vi "Request Data.vi"(6 "Qualifier":string, 8 "error in":errorcluster, 9 "notifier":refnum<notifier>, 10 "Data to Send":string, 11 "Analog-Output in":refnum<class "Analog-Output.lvclass">) -> (0 "error out":errorcluster, 3 "Analog-Output out":refnum<class "Analog-Output.lvclass">)   [LabVIEW 2019, in "Analog-Output.lvlib" / "Analog-Output.lvclass"]
doc: "Data to Send is a required input that describes the measurement or query function to be performed\nQualifier is a secondary variable used in the event that specificity must be provided to the query function\n****Note****\nIf further specificity is required, the qualifier must be used in a comma delimited format to increase the overall variable count. Additional specificity must be provided by the child class and interpreted by the automated call.\n\nnotifier is a single variant notifier in which the instrument will send the data notification to the automated tool."
uses:
  Library/Analog-Output.lvclass
  C:/Users/Public/Documents/Development/builds/Engine/Monitored Actor.lvlibp/Monitored Actor/Monitored Actor/Monitored Actor.lvclass
  C:/Users/Public/Documents/Development/builds/Instruments/Instruments.lvlibp/Library/Instruments.lvclass
  Library/Analog-Output.lvclass/Analog-Output.ctl
  <vilib>/Utility/error.llb/Error Cluster From Error Code.vi
  builds/Engine/Monitored Actor.lvlibp/Monitored Actor/Monitored Actor/Read Actor Label.vi
  builds/Instruments/Instruments.lvlibp/Private/Accessors/Read Poll(ms).vi
  builds/Instruments/Instruments.lvlibp/Private/Polymorphic/Special/Event from String.vi
  builds/Instruments/Instruments.lvlibp/Accessors/Command with Logging.vi
  <vilib>/ErrorRing/Error Ring.xnode
  builds/Instruments/Instruments.lvlibp/Library/Instruments.lvclass
  builds/Instruments/Instruments.lvlibp
  builds/Engine/Engine.lvlibp/Project/Engine.lvclass
  C:/Users/Public/Documents/Development/builds/Engine/Engine.lvlibp/Project/Engine.lvclass
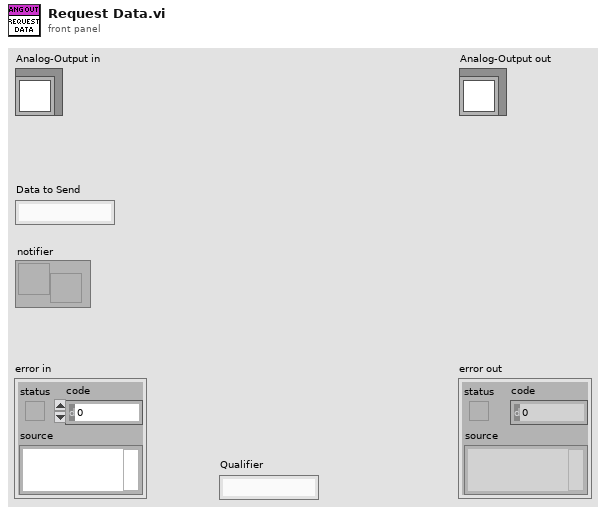
[diagram p1: front panel]
types:
  T1 = cluster{"Timestamp":timestamp, "Description":string, "Data":string}
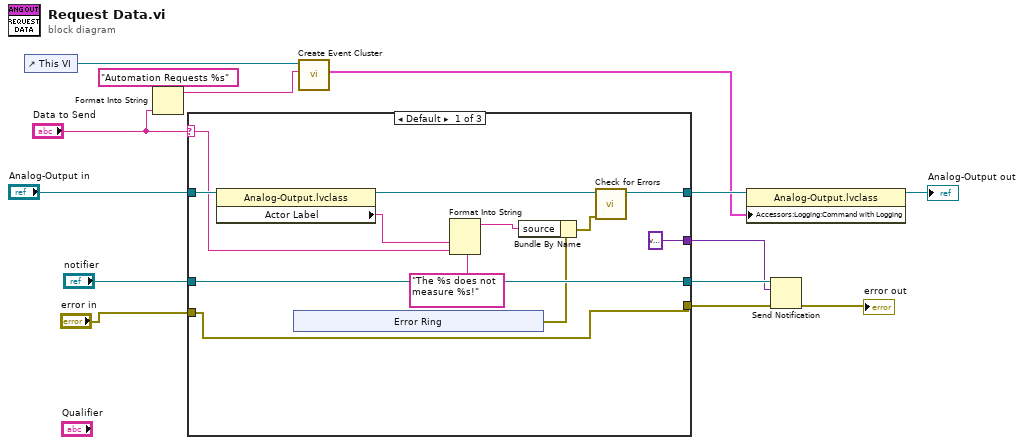
[diagram p0: block diagram]
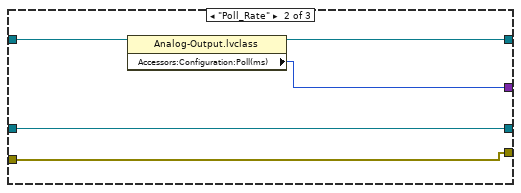
[diagram p2: hidden frame]
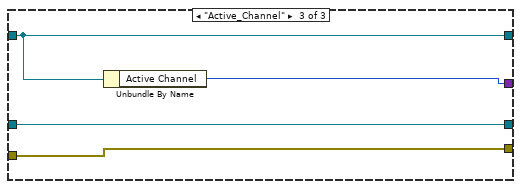
[diagram p3: hidden frame]
diagram:
  n1 = control-ref of="This VI"() -> (w11:refnum<vi>)
  n2 = Format Into String(format string="Automation Requests %s", "Data to Send") -> (resulting string=w8:string)  [unwired: 2 in, 1 out]
  n3 = case shown="Default" "Data to Send" {
    selector: "Data to Send" -> [w24 _ _]
    tunnel: "Analog-Output in" -> [w25 w35 w38]
    tunnel: [w26 w31 w39] -> w13
    tunnel: "notifier" -> [w26 w31 w39]
    tunnel: [w20 w33 w38] -> w7
    tunnel: "error in" -> [w18 w32 w37]
    tunnel: [w18 w32 w37] -> w3
    tunnel: [variant w34 w36] -> w2
    frame Default {
      n4 = property class="Analog-Output.lvclass"(reference=w25) -> (reference out=w21:refnum<class "Analog-Output.lvclass">, "Actor Label"=w23:string)  [unwired: 1 in, 1 out]
      n5 = xnode "Error Ring"() -> ("error out"=w15:errorcluster)
      n6 = Format Into String(format string="The %s does not measure %s!", w23, w24) -> (resulting string=w16:string)  [unwired: 2 in, 1 out]
      n7 = Bundle By Name(cluster=w15, "source"=w16) -> (w17:errorcluster)
      n8 = call "Check for Errors.vi"("error in"=w17, "Engine in"=w21) -> ("Engine out"=w20:refnum<class "Analog-Output.lvclass">)  [unwired: 8 in, 1 out]
    }
    frame "Poll_Rate" {
      n9 = property class="Analog-Output.lvclass"(reference=w35) -> (reference out=w33:refnum<class "Analog-Output.lvclass">, "Accessors:Configuration:Poll(ms)"=w34:u32)  [unwired: 1 in, 1 out]
    }
    frame "Active_Channel" {
      n10 = Unbundle By Name(w38) -> ("Active Channel"=w36:u32)
    }
  }
  n11 = call-poly "Create Event Cluster.vi"("Value"=w8, "VI Refnum"=w11) -> ("Event Data"=w6:T1)  [unwired: 9 in]
  n12 = property class="Analog-Output.lvclass"(reference=w7, "Accessors:Logging:Command with Logging"=w6) -> (reference out=→"Analog-Output out":refnum<class "Analog-Output.lvclass">)  [unwired: 1 in, 1 out]
  n13 = Send Notification(notification=w2, notifier=w13, error in (no error)=w3) -> (error out=→"error out":errorcluster)  [unwired: 1 out]
